vi "Reading Green.vi"() -> ()   [LabVIEW 2022 SP3]
panel:
  in  "Numeric":dbl
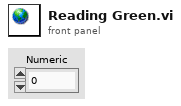
[diagram p1: front panel]
diagram:
